vi "Variant To JSON.vi"(8 "error in (no error)":errorcluster, 10 "Variant":variant) -> (0 "error out":errorcluster, 3 "JSON Value out":refnum<class "JSON Value.lvclass">)   [LabVIEW 2016, in "JSFL Variant Support.lvlib"]
doc: "Creates a new JSON instance of the given type specified by the variant."
uses:
  JSFL Variant Support.lvlib
  JSON Value.lvclass
  New JSON Value/New JSON (String).vi
  <vilib>/Utility/Data Type/NI_Data Type.lvlib
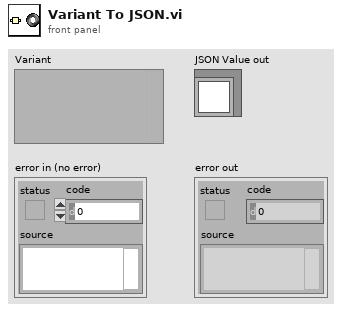
[diagram p1: front panel]
types:
  T1 = typedef "NI_Data Type.lvlib/Data Type.ctl" = enum8{"Invalid Type", "Void", "I8", "I16", "I32", "I64", "U8", "U16", "U32", "U64", "Single Float", "Double Float", "Extended Float", "Single Complex", "Double Complex", "Extended Complex", "Enum U8", "Enum U16", "Enum U32", "Enum U64", "Single Float With Unit", "Double Float With Unit", "Extended Float With Unit", "Single Complex with Unit", "Double Complex with Unit", "Extended Complex with Unit", "Boolean", "String", "Path", "Picture", "Tag", "Array", "Cluster", "Variant", "LV Variant", "Waveform", "Timestamp", "Digital Waveform", "Digital Data", "ExpressData", "Refnum", "External Data", "VI", "Poly VI", "LabVIEW Class Instance", "Fixed Point"}
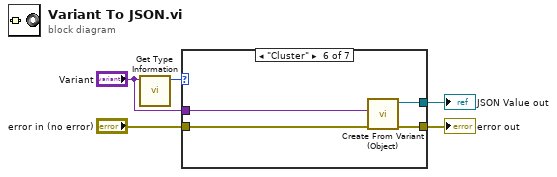
[diagram p0: block diagram]
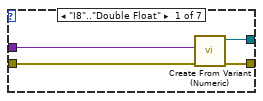
[diagram p2: hidden frame]
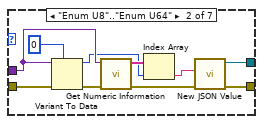
[diagram p3: hidden frame]
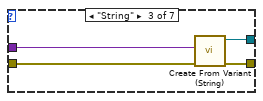
[diagram p4: hidden frame]
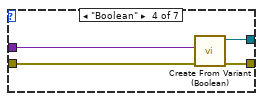
[diagram p5: hidden frame]
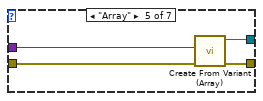
[diagram p6: hidden frame]
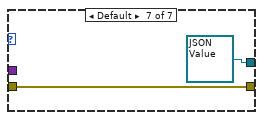
[diagram p7: hidden frame]
diagram:
  n1 = call <vilib>:"Get Type Information.vi"("Variant"="Variant") -> ("Type"=w5:T1)  [unwired: 6 in, 4 out]
  n2 = case shown="\"Cluster\"" w5 {
    tunnel: "Variant" -> [w9 w17 w20 w27 w31 w35 _]
    tunnel: [w6 w19 w23 w24 w30 w32 refnum<class "JSON Value.lvclass"> refnum ("JSON out")] -> w1
    tunnel: "error in (no error)" -> [w8 w12 w21 w26 w29 w34 w37]
    tunnel: [w7 w18 w22 w25 w28 w33 w37] -> w2
    frame "I8".."Double Float" {
      n3 = call "Create From Variant (Numeric).vi"("error in (no error)"=w8, "Variant"=w9) -> ("error out"=w7:errorcluster, "JSON Value out"=w6:refnum<class "JSON Value.lvclass">)  [unwired: 8 in]
    }
    frame "Enum U8".."Enum U64" {
      n4 = Variant To Data(error in=w12, type=u64 0, Variant=w17) -> (data=w14:u64, error out=w11:errorcluster)
      n5 = call <vilib>:"Get Numeric Information.vi"("error in (no error)"=w11, "Variant"=w17) -> ("error out"=w10:errorcluster, "Enum Names"=w15:string[])  [unwired: 6 in, 2 out]
      n6 = Index Array(array=w15, index=w14) -> (element=w13:string)
      n7 = call-poly "New JSON Value.vi"("error in (no error)"=w10, "value"=w13) -> ("error out"=w18:errorcluster, "JSON Value out"=w19:refnum<class "JSON Value.lvclass">)  [unwired: 8 in]
    }
    frame "String" {
      n8 = call "Create From Variant (String).vi"("error in (no error)"=w21, "Variant"=w20) -> ("error out"=w22:errorcluster, "JSON Value out"=w23:refnum<class "JSON Value.lvclass">)  [unwired: 8 in]
    }
    frame "Boolean" {
      n9 = call "Create From Variant (Boolean).vi"("error in (no error)"=w26, "Variant"=w27) -> ("error out"=w25:errorcluster, "JSON Value out"=w24:refnum<class "JSON Value.lvclass">)  [unwired: 8 in]
    }
    frame "Array" {
      n10 = call "Create From Variant (Array).vi"("error in (no error)"=w29, "Variant"=w31) -> ("error out"=w28:errorcluster, "JSON Value out"=w30:refnum<class "JSON Value.lvclass">)  [unwired: 8 in]
    }
    frame "Cluster" {
      n11 = call "Create From Variant (Object).vi"("error in (no error)"=w34, "Variant"=w35) -> ("error out"=w33:errorcluster, "JSON Value out"=w32:refnum<class "JSON Value.lvclass">)  [unwired: 8 in]
    }
    frame Default {
    }
  }
  "error out" <- w2
  "JSON Value out" <- w1
